vi "solar_excel Cell String to Range.vi"(11 "Cell String ('A1')":string) -> (3 "Range":cluster{"Row":u32, "Column":u32})   [LabVIEW 2018]
doc: "This converts an Excel range (i.e. 'B3') into a row & column pair. Ex: 'C4' = Col:3, Row:4"
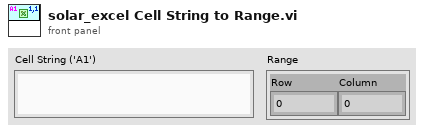
[diagram p1: front panel]
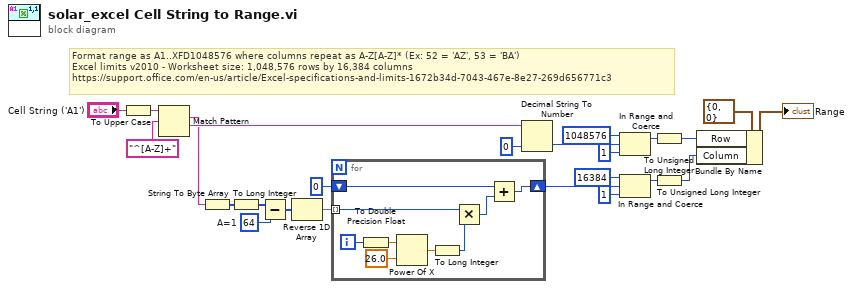
[diagram p0: block diagram]
diagram:
  w15 = 64  # A=1
  # "Format range as A1..XFD1048576 where columns repeat as A-Z[A-Z]* (Ex: 52 = 'AZ', 53 = 'BA')\nExcel limits v2010 - Worksheet size: 1,048,576 rows by 16,384 columns\nhttps://support.office.com/en-us/article/Excel-specifications-and-limits-1672b34d-7043-467e-8e27-269d656771c3"
  n1 = To Upper Case(1:"Cell String ('A1')") -> (0:w22:string)
  n2 = Match Pattern(string=w22, regular expression="^[A-Z]+") -> (match substring=w17:string, after substring=w21:string)  [unwired: 1 in, 2 out]
  n3 = String To Byte Array(string=w17) -> (unsigned byte array=w16:u8[])
  n4 = To Long Integer(number=w16) -> (32bit integer=w13:i32[])
  n5 = Subtract(x=w13, y=w15) -> (x-y=w14:i32[])
  n6 = Reverse 1D Array(array=w14) -> (reversed array=w12:i32[])
  n7 = for {
    tunnel: w12 -> [w29] mode=indexing
    shift-right: [w26] -> w5
    shift-left: 0 -> [w25]
    i -> [w33]
    n8 = To Double Precision Float(number=w33) -> (double precision float=w32:dbl)
    n9 = Power Of X(1:26.0 ("x"), 2:w32) -> (0:w30:dbl)
    n10 = To Long Integer(number=w30) -> (32bit integer=w28:i32)
    n11 = Multiply(x=w29, y=w28) -> (x*y=w27:i32)
    n12 = Add(x=w25, y=w27) -> (x+y=w26:i32)
  }
  n13 = Decimal String To Number(string=w21, default (0L)=0 ("default (0 I32)")) -> (number=w10:i32)  [unwired: 1 in, 1 out]
  n14 = In Range and Coerce(upper limit=1048576, x=w10, lower limit=1) -> (coerced(x)=w3:i32)  [unwired: 1 out]
  n15 = In Range and Coerce(upper limit=16384, x=w5, lower limit=1) -> (coerced(x)=w4:i32)  [unwired: 1 out]
  n16 = To Unsigned Long Integer(number=w3) -> (unsigned 32bit integer=w1:u32)
  n17 = To Unsigned Long Integer(number=w4) -> (unsigned 32bit integer=w2:u32)
  n18 = Bundle By Name(cluster=cluster{"Row":u32, "Column":u32} {"Row"=0, "Column"=0} ("Range"), "Row"=w1, "Column"=w2) -> (→"Range":cluster{"Row":u32, "Column":u32})
